vi "toggle_ctrls_by_label.vi"(6 "States":bool[](array[boolean]), 7 "Names":string[](array[string]), 8 "error in":errorcluster, 9 "Boolean in":refnum<vi>) -> (0 "error out":errorcluster, 1 "Boolean out":refnum<vi>)   [LabVIEW 2016]
uses:
  <userlib>/_OpenG.lib/array/array.llb/Filter 1D Array (String)__ogtk.vi
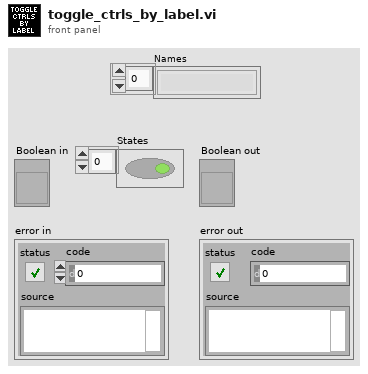
[diagram p1: front panel]
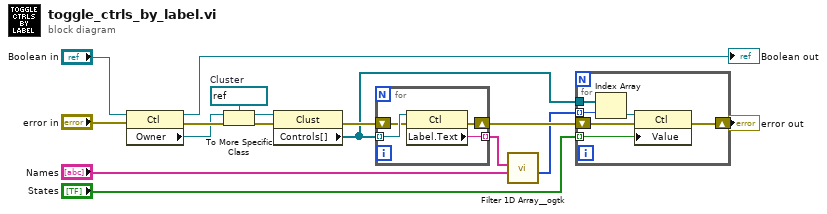
[diagram p0: block diagram]
diagram:
  w11 = refnum<vi> refnum  # Cluster
  n1 = property class="Ctl"(reference="Boolean in", error in="error in") -> (reference out=→"Boolean out":refnum<vi>, error out=w13:errorcluster, "Owner"=w12:refnum<vi>)
  n2 = To More Specific Class(target class=w11, reference=w12, error in=w13) -> (specific class reference=w10:refnum<vi>, error out=w9:errorcluster)
  n3 = property class="Clust"(reference=w10, error in=w9) -> (error out=w8:errorcluster, "Controls[]"=w6:refnum<vi>[])  [unwired: 1 out]
  n4 = for {
    tunnel: w6 -> [w20] mode=indexing
    tunnel: [w18] -> w7 mode=indexing
    shift-right: [w17] -> w4
    shift-left: w8 -> [w19]
    n5 = property class="Ctl"(reference=w20, error in=w19) -> (error out=w17:errorcluster, "Label.Text"=w18:string)  [unwired: 1 out]
  }
  n6 = call-poly <userlib>:"Filter 1D Array__ogtk.vi"("items to filter"="Names", "array"=w7) -> ("filtered item indices"=w2:i32[])  [unwired: 4 in, 1 out]
  n7 = for {
    tunnel: w2 -> [w25] mode=indexing
    tunnel: w6 -> [w26]
    shift-right: [w22] -> w3
    shift-left: w4 -> [w23]
    tunnel: "States" -> [w21] mode=indexing
    n8 = Index Array(array=w26, index=w25) -> (element=w24:refnum<vi>)
    n9 = property class="Ctl"(reference=w24, error in=w23, "Value"=w21) -> (error out=w22:errorcluster)  [unwired: 1 out]
  }
  "error out" <- w3
